vi "Get Library Class Name.vi"(11 "VI In":string) -> (0 "Found?":bool, 3 "Name":string)   [LabVIEW 2020, in "SimpleDependencyInspector.lvlib"]
uses:
  SimpleDependencyInspector.lvlib
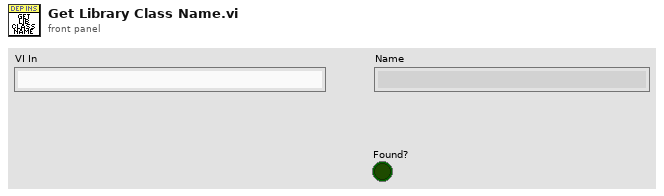
[diagram p1: front panel]
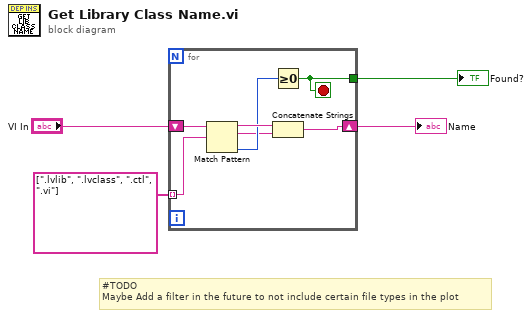
[diagram p0: block diagram]
diagram:
  # "#TODO\nMaybe Add a filter in the future to not include certain file types in the plot"
  n1 = for {
    tunnel: string[] [".lvlib", ".lvclass", ".ctl", ".vi"] ("regular expression") -> [w6] mode=indexing
    shift-right: [w7] -> w1
    shift-left: "VI In" -> [w11]
    tunnel: [w8] -> w2
    stop <- w8 stop-if-true
    n2 = Match Pattern(string=w11, regular expression=w6) -> (before substring=w10:string, match substring=w5:string, offset past match=w9:i32)  [unwired: 1 in, 1 out]
    n3 = Greater Or Equal To 0?(x=w9) -> (x >= 0?=w8:bool)
    n4 = Concatenate Strings(w10, w5) -> (w7:string)
  }
  "Name" <- w1
  "Found?" <- w2
